vi "START_SESSION_DECODE.vi"(6 "MIMIC HOST COMMAND":T2(ring)=enum."Start Session", 8 "Input String Data Array":string[](array[string])=["1"], 9 "HWHSflag":bool, 10 "wait (ms)":u32=500, 11 "VISA resource name":refnum<visa-resource-name>="COM6") -> (0 "error out":errorcluster={"status"=FALSE, "code"=1073676294, "source"="VISA Read in MIMIC RecvCommand.vi->MIMIC Commands Rev 2.vi"}, 1 "Receive_buffer":u8[](array[numeric]) format="%x", 2 "Receive_Unpacked_Data":T1)   [LabVIEW 2014]
panel:
  out "local":i32
  out "GUID":string
  out "Array":u8[](array[numeric]) format="%x"
  out "TimeToDecode":u16
  out "VISA resource name OUT":refnum<visa-resource-name>="COM6"
  out "hex integer string":string[](array[string])=["4", "D0", "0", "0", "FF", "2C"]
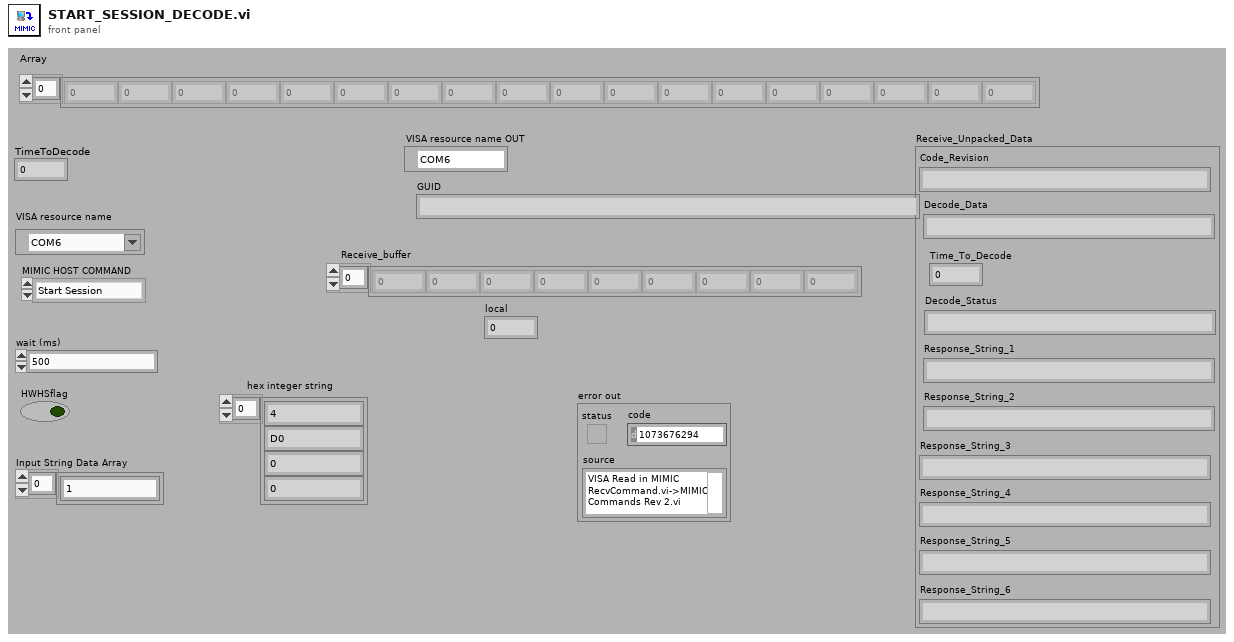
[diagram p1: front panel]
types:
  T1 = cluster{"Code_Revision":string, "Decode_Data":string, "Decode_Status":string, "Response_String_1":string, "Response_String_2":string, "Response_String_3":string, "Response_String_4":string, "Response_String_5":string, "Response_String_6":string, "Time_To_Decode":u16}
  T2 = enum16{"Enter FAT", "Beeper Control", "LED Off", "LED On", "Image Mode", "Start Session", "Stop Session", "Change Buadrate", "Auto Exposure", "Set Manual Exposure", "Read BT Address", "Store BT Address", "Pairing Command", "Query Paired Address", "Pairing Status", "Un-Pairing", "Set Illumination", "Trigger", "Set Defaults", "Imager Time To Decode Test", "Battery Off", "Battery Charge Control", "Read Battery Voltage", "Read Battery Temperature", "Software Version", "StoreFeatureSet", "ReadFeatureSet", "Store Model Number", "Read Model Number", "Store Manufacturing Date", "Read Manufacturing Date", "Store Service Date", "Read Service Date", "Store Serial Number", "Read Serial Number", "Exit FAT", "Read GUID", "Cable Auto ID", "Store RSM 627", "Read RSM 627", "Hall Effect switch", "Store GUID ", "ParamSend", "General", "General-Response", "RSM Init", "RSM EnterFAT", "RSM - SE4500 - Peek PRISM Register GENERIC command", "RSM - SE4500 - Poke PRISM Register GENERIC command", "RSM - SE4500 - GENERIC command", "RSM - SE4500 - GetPDM Calibration", "RSM - SE4500 - SetPDM Calibration", "Get Object Sensor Value", "Store Object Sensor Calibration Value", "Read Object Sensor Calibration Value", "RSM - SE4500 - GetPDM-Z Calibration", "RSM - SE4500 - SetPDM-Z Calibration"}
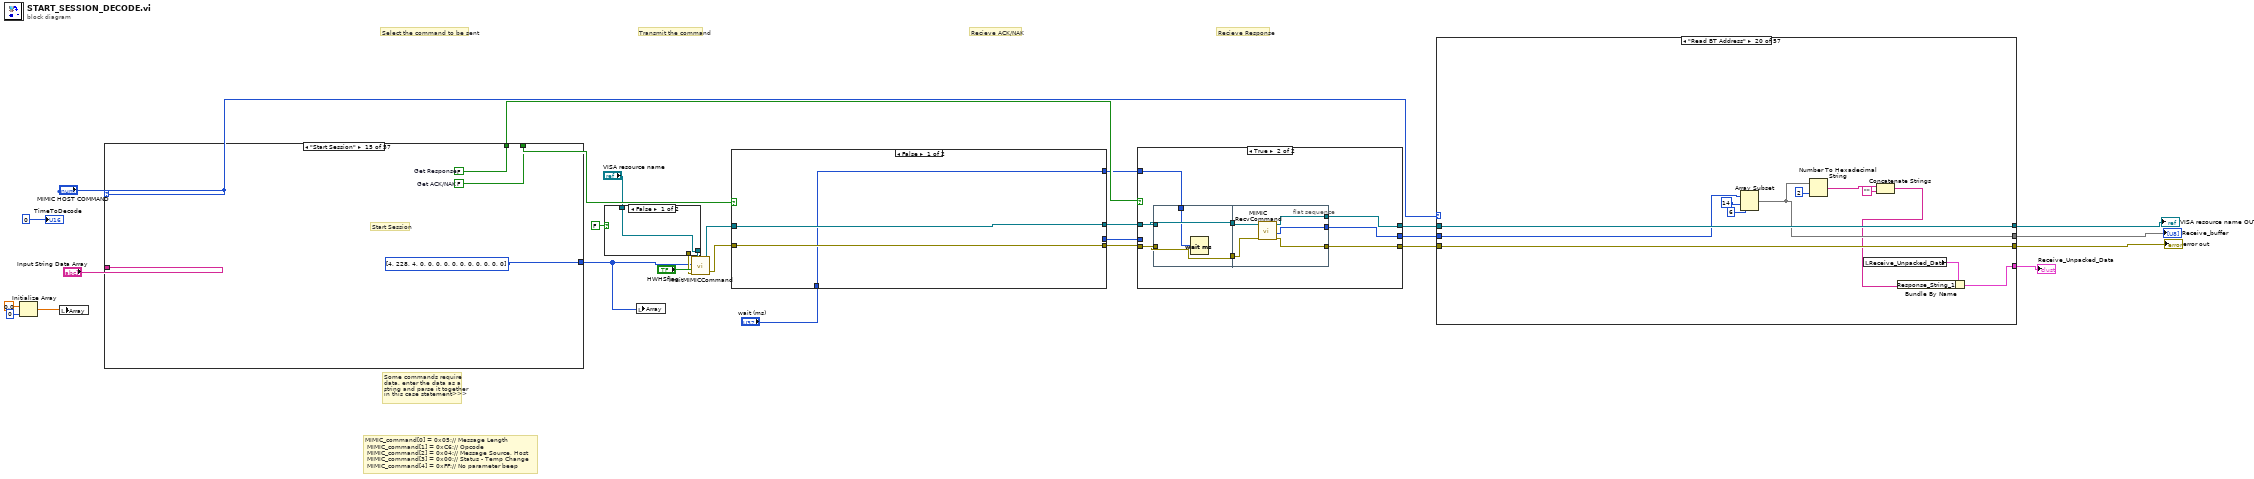
[diagram p0: block diagram]
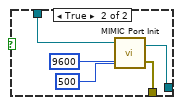
[diagram p2: hidden frame]
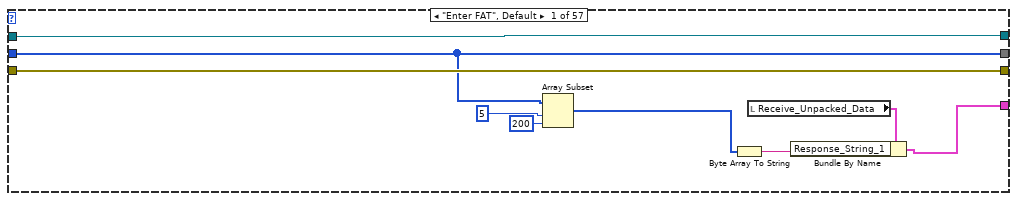
[diagram p3: hidden frame]
diagram:
  # "MIMIC_command[0] = 0x05;// Message Length \n\tMIMIC_command[1] = 0xC6;// Opcode  \n\tMIMIC_command[2] = 0x04;// Message Source, Host \n\tMIMIC_command[3] = 0x00;// Status - Temp Change            \n\tMIMIC_command[4] = 0xFF;// No parameter beep"
  # "Transmit the command"
  # "Recieve Response"
  # "Recieve ACK/NAK"
  # "Select the command to be sent"
  # "Some commands require\ndata, enter the data as a\nstring and parse it together\nin this case statement>>>"
  n1 = Initialize Array(0.0 ("element"), 0 ("dimension size")) -> (w5:dbl[])
  n2 = local write "Array"(w5) -> ()
  n3 = case shown="\"Start Session\"" "MIMIC HOST COMMAND" {
    tunnel: "Input String Data Array" -> [w37 w39 w62 _ _ _ _ _ w86 w113 w139 w179 w219 w256 _ _ _ w274 w290 w300 w313 w331 w347 _ _ _ _ _ w371 _ _ _ w391 _ _ _ _ w416 _ w428 _ w438 _ _ _ w464 _ w476 _ _ _ _ _ _ _ _ _]
    tunnel: [w31 w45 w66 u8[] [5, 161, 4, 128, 16, 0, 0, 0, 0, 0, 0, 0, 0, 0] u8[] [14, 128, 4, 0, 0, 10, 112, 0, 1, 20, 112, 12, 0, 132] u8[] [14, 128, 4, 0, 0, 10, 112, 0, 1, 20, 112, 31, 0, 113] u8[] [12, 128, 4, 0, 0, 6, 32, 0, 0, 240, 0, 0, 0, 0] u8[] [13, 128, 4, 0, 0, 9, 112, 0, 1, 2, 120, 1, 135, 0] w85 w119 w140 w176 w217 w257 u8[] [4, 228, 4, 0, 0, 0, 0, 0, 0, 0, 0, 0, 0, 0] u8[] [4, 228, 4, 0, 0, 0, 0, 0, 0, 0, 0, 0, 0, 0] u8[] [7, 215, 4, 0, 4, 11, 0, 255, 15, 0, 0, 0, 0, 0] w275 w284 w298 w317 w334 w346 u8[] [16, 161, 4, 128, 16, 0, 0, 0, 0, 0, 0, 0, 0, 0] u8[] [5, 161, 4, 128, 16, 0, 0, 0, 0, 0, 0, 0, 0, 0] u8[] [4, 200, 4, 128, 0, 0, 0, 0, 0, 0, 0, 0, 0, 0] u8[] [5, 161, 4, 128, 25, 0, 0, 0, 0, 0, 0, 0, 0, 0] u8[] [7, 161, 4, 128, 66, 2, 29, 0, 0, 0, 0, 0, 0, 0] w370 u8[] [6, 161, 4, 128, 45, 2, 0, 0, 0, 0, 0, 0, 0, 0] u8[] [7, 161, 4, 128, 48, 19, 136, 0, 0, 0, 0, 0, 0, 0] u8[] [5, 161, 4, 128, 60, 0, 0, 0, 0, 0, 0, 0, 0, 0] w390 u8[] [7, 161, 4, 128, 66, 117, 48, 0, 0, 0, 0, 0, 0, 0] u8[] [7, 161, 4, 128, 66, 117, 49, 0, 0, 0, 0, 0, 0, 0] u8[] [7, 161, 4, 128, 66, 78, 41, 0, 0, 0, 0, 0, 0, 0] u8[] [6, 161, 4, 128, 96, 8] w409 u8[] [7, 161, 4, 128, 66, 3, 36] w430 u8[] [7, 161, 4, 128, 66, 2, 194, 0, 0, 0, 0, 0, 0, 0] w443 u8[] [7, 161, 4, 128, 66, 2, 21, 0, 0, 0, 0, 0, 0, 0] w457 u8[] [7, 161, 4, 128, 66, 2, 23, 0, 0, 0, 0, 0, 0, 0] w469 u8[] [7, 161, 4, 128, 66, 2, 24, 0, 0, 0, 0, 0, 0, 0] w481 u8[] [7, 161, 4, 128, 66, 2, 22, 0, 0, 0, 0, 0, 0, 0] u8[] [5, 161, 4, 128, 54, 254, 160, 0, 0, 0, 0, 0, 0, 0] u8[] [5, 161, 4, 128, 84, 0, 0, 0, 0, 0, 0, 0, 0, 0] u8[] [5, 161, 4, 128, 47] w496 u8[] [5, 161, 4, 128, 110] u8[] [10, 161, 4, 128, 69, 2, 115, 66, 7, 2] u8[] [6, 161, 4, 128, 45, 1, 0, 0, 0, 0, 0, 0, 0, 0] u8[] [7, 161, 4, 128, 66, 2, 115]] -> w6
    tunnel: [w30 w57 w64 w71 w75 w78 w81 w84 w108 w135 w172 w192 w232 w258 w266 w269 w271 w276 w291 w301 w318 w335 w353 w356 w358 w361 w365 w369 w373 w380 w384 w387 w388 w399 w402 w404 w407 w422 w425 w433 w436 w442 w447 w456 w461 w468 w472 w479 w484 w488 w492 w493 w501 w503 w506 w509 w513] -> w25
    tunnel: [w29 w56 w65 w70 w74 w77 w80 w83 w107 w134 w171 w191 w231 w259 w267 w270 w272 w277 w292 w302 w319 w336 w354 w357 w359 w362 w364 w368 w372 w381 w383 w386 w389 w398 w401 w403 w406 w421 w424 w432 w435 w441 w448 w455 w460 w467 w473 w480 w485 w487 w491 w494 w502 w504 w507 w510 w512] -> w27
    frame "LED On" {
      w30 = FALSE  # Get Response
      w29 = TRUE  # Get ACK/NAK
      # "LED data Byte"
      n4 = Index Array(array=w37, index=0) -> (element=w36:string)
      n5 = Decimal String To Number(string=w36) -> (number=w35:i32)  [unwired: 2 in, 1 out]
      n6 = Replace Array Subset(array=u8[] [5, 231, 4, 128, 1, 0, 0, 0, 0, 0, 0, 0, 0, 0], new element=w35, index=4) -> (w31:u8[])
    }
    frame "ParamSend" {
      w57 = FALSE  # Get Response
      w56 = TRUE  # Get ACK/NAK
      n7 = Array Size(array=w39) -> (size(s)=w38:i32)
      n8 = Index Array(array=w39, index=0) -> (element=w61:string)
      n9 = Add(x=w38, y=5) -> (x+y=w43:i32)
      n10 = Hexadecimal String To Number(string=w61) -> (number=w42:u32)  [unwired: 2 in, 1 out]
      n11 = Replace Array Subset(array=u8[] [5, 198, 4, 128, 255, 0, 0, 0, 0, 0, 0, 0, 0, 0], new element=w43, index=0) -> (w54:u8[])
      n12 = Replace Array Subset(array=w54, new element=w42, index=5) -> (w50:u8[])
      n13 = Index Array(array=w39, index=2) -> (element=w49:string)
      n14 = Index Array(array=w39, index=1) -> (element=w53:string)
      n15 = Hexadecimal String To Number(string=w49) -> (number=w40:u32)  [unwired: 2 in, 1 out]
      n16 = Hexadecimal String To Number(string=w53) -> (number=w41:u32)  [unwired: 2 in, 1 out]
      n17 = Replace Array Subset(array=w50, new element=w41, index=6) -> (w46:u8[])
      n18 = Replace Array Subset(array=w46, new element=w40, index=7) -> (w45:u8[])
    }
    frame "Beeper Control" {
      w64 = FALSE  # Get Response
      w65 = TRUE  # Get ACK/NAK
      # "Beeper data Byte"
      n19 = Decimal String To Number(string=w62, offset=0) -> (number=w69:i32[])  [unwired: 1 in, 1 out]
      n20 = Replace Array Subset(array=u8[] [5, 230, 4, 128, 0, 0, 0, 0, 0, 0, 0, 0, 0, 0], new element=w69, index=4) -> (w66:u8[])
    }
    frame "Enter FAT" {
      w71 = TRUE  # Get Response
      w70 = TRUE  # Get ACK/NAK
      # "Enter FAT command:\n0x05:0xA1:0x40:0x80:0x10"
    }
    frame "RSM - SE4500 - GetPDM Calibration" {
      w75 = TRUE  # Get Response
      w74 = FALSE  # Get ACK/NAK
      # "RSM GetDPMCalibration Command"
    }
    frame "RSM - SE4500 - GetPDM-Z Calibration" {
      w78 = TRUE  # Get Response
      w77 = FALSE  # Get ACK/NAK
      # "RSM GetDPMCalibration Command"
    }
    frame "RSM Init" {
      w81 = TRUE  # Get Response
      w80 = FALSE  # Get ACK/NAK
      # "Init RSM command:\n0x0C:0x80:0x04:0x00:0x00:0x06:0x20:0x00:0x00:0xF0"
    }
    frame "RSM EnterFAT" {
      w84 = TRUE  # Get Response
      w83 = FALSE  # Get ACK/NAK
      # "RSM / SE4500 - Enter FAT command:\n0x0D:0x80:0x04:0x00:0x00:0x09:0x70:0x00:0x01:0x02:0x78:0x01:0x87:"
    }
    frame "RSM - SE4500 - Peek PRISM Register GENERIC command" {
      w108 = TRUE  # Get Response
      w107 = FALSE  # Get ACK/NAK
      # "Register Word - HEX String"
      # "RSM / SE4500 - Peek PRISM Register GENERIC command:\n0x0E:0x80:0x04:0x00:0x00:0x0B:0x70:0x00:0x01:0x02:0xC3:0xXX:0xXX:0xXX:0xCS"
      n21 = Index Array(array=w86, index=0) -> (element=w90:string)
      n22 = Hexadecimal String To Number(string=w90, default (0uL)=i16 0 ("default (0 I32)")) -> (number=w88:i16)  [unwired: 1 in, 1 out]
      n23 = Split Number(x=w88) -> (hi(x)=w94:u8, lo(x)=w92:u8)
      n24 = Replace Array Subset(array=u8[] [15, 128, 4, 0, 0, 11, 112, 0, 1, 3, 195, 0, 0, 0, 0], new element=w94, index=11) -> (w91:u8[])
      n25 = Replace Array Subset(array=w91, new element=w92, index=12) -> (w87:u8[])
      n26 = Array Subset(array=w87, index=10, length=3) -> (w97:u8[])
      n27 = for {
        N: 3 -> [_]
        tunnel: w97 -> [w111] mode=indexing
        shift-right: [w109] -> w103
        shift-left: u16 0 -> [w110]
        n28 = Add(x=w110, y=w111) -> (x+y=w109:u16)
      }
      n29 = Not(x=w103) -> (.not. x?=w102:u16)
      n30 = Increment(x=w102) -> (x+1=w101:u16)
      n31 = Replace Array Subset(array=w87, new element=w101, index=13) -> (w85:u8[])
    }
    frame "RSM - SE4500 - GENERIC command" {
      w114 = 1 ("index")
      w118 = 0 ("index")
      w135 = TRUE  # Get Response
      w134 = FALSE  # Get ACK/NAK
      # "Register Word - HEX String"
      # "RSM / SE4500 - Peek PRISM Register GENERIC command:\n0x0E:0x80:0x04:0x00:0x00:0x0B:0x70:0x00:0x01:0x02:0xXX:0xXX:0xXX:0xCS"
      n32 = Index Array(array=w113, index=w118) -> (element=w121:string)
      n33 = Index Array(array=w113, index=w114) -> (element=w115:string)
      n34 = Hexadecimal String To Number(string=w121, default (0uL)=w118) -> (number=w116:i32)  [unwired: 1 in, 1 out]
      n35 = Hexadecimal String To Number(string=w115, default (0uL)=w114) -> (number=w112:i32)  [unwired: 1 in, 1 out]
      n36 = Replace Array Subset(array=u8[] [13, 128, 4, 0, 0, 9, 112, 0, 1, 2, 255, 0, 0], new element=w116, index=10) -> (w122:u8[])
      n37 = Replace Array Subset(array=w122, new element=w112, index=11) -> (w120:u8[])
      n38 = Array Subset(array=w120, index=10, length=2) -> (w125:u8[])
      n39 = for {
        N: 2 -> [_]
        tunnel: w125 -> [w138] mode=indexing
        shift-right: [w136] -> w131
        shift-left: u16 0 -> [w137]
        n40 = Add(x=w137, y=w138) -> (x+y=w136:u16)
      }
      n41 = Not(x=w131) -> (.not. x?=w130:u16)
      n42 = Increment(x=w130) -> (x+1=w129:u16)
      n43 = Replace Array Subset(array=w120, new element=w129, index=12) -> (w119:u8[])
    }
    frame "RSM - SE4500 - Poke PRISM Register GENERIC command" {
      w172 = TRUE  # Get Response
      w171 = FALSE  # Get ACK/NAK
      # "Register Word - HEX String"
      # "Register Word - HEX String"
      # "Value Byte - Decimal String"
      # "RSM / SE4500 - Poke PRISM Register GENERIC command:\n0x0E:0x80:0x04:0x00:0x00:0x0B:0x70:0x00:0x01:0x02:0xC0:0xXX:0xXX:0xXX:0xCS"
      n44 = Index Array(array=w139, index=0) -> (element=w154:string)
      n45 = Index Array(array=w139, index=1) -> (element=w145:string)
      n46 = Hexadecimal String To Number(string=w154, default (0uL)=i16 0 ("default (0 I32)")) -> (number=w152:i16)  [unwired: 1 in, 1 out]
      n47 = Split Number(x=w152) -> (hi(x)=w158:u8, lo(x)=w156:u8)
      n48 = Hexadecimal String To Number(string=w145, default (0uL)=i16 0 ("default (0 I32)")) -> (number=w151:i16)  [unwired: 1 in, 1 out]
      n49 = Replace Array Subset(array=u8[] [16, 128, 4, 0, 0, 12, 112, 0, 1, 2, 151, 0, 0, 0, 0, 0], new element=w158, index=12) -> (w155:u8[])
      n50 = Split Number(x=w151) -> (hi(x)=w148:u8, lo(x)=w150:u8)
      n51 = Replace Array Subset(array=w155, new element=w156, index=11) -> (w143:u8[])
      n52 = Replace Array Subset(array=w143, new element=w148, index=14) -> (w142:u8[])
      n53 = Replace Array Subset(array=w142, new element=w150, index=13) -> (w141:u8[])
      n54 = Array Subset(array=w141, index=10, length=5) -> (w161:u8[])
      n55 = for {
        N: 5 -> [_]
        tunnel: w161 -> [w175] mode=indexing
        shift-right: [w173] -> w167
        shift-left: u16 0 -> [w174]
        n56 = Add(x=w174, y=w175) -> (x+y=w173:u16)
      }
      n57 = Not(x=w167) -> (.not. x?=w166:u16)
      n58 = Increment(x=w166) -> (x+1=w165:u16)
      n59 = Replace Array Subset(array=w141, new element=w165, index=15) -> (w140:u8[])
    }
    frame "RSM - SE4500 - SetPDM Calibration" {
      w192 = TRUE  # Get Response
      w191 = FALSE  # Get ACK/NAK
      # "RSM / SE4500 - SetDPMCalibration command:"
      n60 = for {
        N: 8 -> [_]
        shift-right: [w202] -> w178
        shift-left: u8[] [30, 128, 4, 0, 0, 26, 112, 0, 1, 2, 148, 12, 0, 0, 0, 0, 0, 0, 0, 0, 0, 0, 0, 0, 0, 0, 0, 0, 0, 0, 0] -> [w209]
        tunnel: w179 -> [w208]
        i -> [w204]
        # "high byte"
        # "low byte"
        n61 = Index Array(array=w208, index=w204) -> (element=w197:string)
        n62 = Decimal String To Number(string=w197, default (0L)=0 ("default (0 I32)")) -> (number=w194:i32)  [unwired: 1 in, 1 out]
        n63 = Number To Hexadecimal String(1:i16 4 ("width (-)"), 2:w194) -> (0:w195:string)
        n64 = local read "local"() -> (w200:i32)
        n65 = Hexadecimal String To Number(string=w195, default (0uL)=i16 0 ("default (0 I32)")) -> (number=w210:i16)  [unwired: 1 in, 1 out]
        n66 = Add(x=1 ("y"), y=w200) -> (x+y=w198:i32)
        n67 = Add(x=w204, y=w198) -> (x+y=w201:i32)
        n68 = Add(x=1 ("index"), y=w201) -> (x+y=w206:i32)
        n69 = Split Number(x=w210) -> (hi(x)=w212:u8, lo(x)=w211:u8)
        n70 = Replace Array Subset(array=w209, new element=w212, index=w206) -> (w203:u8[])
        n71 = local write "local"(w198) -> ()
        n72 = Replace Array Subset(array=w203, new element=w211, index=w201) -> (w202:u8[])
      }
      n73 = Array Subset(array=w178, index=10, length=19) -> (w182:u8[])
      n74 = for {
        N: 19 -> [_]
        tunnel: w182 -> [w215] mode=indexing
        shift-right: [w213] -> w188
        shift-left: u16 0 -> [w214]
        n75 = Add(x=w214, y=w215) -> (x+y=w213:u16)
      }
      n76 = Not(x=w188) -> (.not. x?=w187:u16)
      n77 = Increment(x=w187) -> (x+1=w186:u16)
      n78 = Replace Array Subset(array=w178, new element=w186, index=29) -> (w176:u8[])
      "local" <- 12 ("x+y")
    }
    frame "RSM - SE4500 - SetPDM-Z Calibration" {
      w232 = TRUE  # Get Response
      w231 = FALSE  # Get ACK/NAK
      # "RSM / SE4500 - SetDPMCalibration command:"
      n79 = local write "local"(12 ("x+y")) -> ()
      n80 = for {
        N: 8 -> [_]
        shift-right: [w242] -> w218
        shift-left: u8[] [30, 128, 4, 0, 0, 26, 112, 0, 1, 2, 148, 31, 0, 0, 0, 0, 0, 0, 0, 0, 0, 0, 0, 0, 0, 0, 0, 0, 0, 0, 0] -> [w249]
        tunnel: w219 -> [w248]
        i -> [w244]
        # "high byte"
        # "low byte"
        n81 = Index Array(array=w248, index=w244) -> (element=w237:string)
        n82 = Decimal String To Number(string=w237, default (0L)=0 ("default (0 I32)")) -> (number=w234:i32)  [unwired: 1 in, 1 out]
        n83 = Number To Hexadecimal String(1:i16 4 ("width (-)"), 2:w234) -> (0:w235:string)
        n84 = local read "local"() -> (w240:i32)
        n85 = Hexadecimal String To Number(string=w235, default (0uL)=i16 0 ("default (0 I32)")) -> (number=w250:i16)  [unwired: 1 in, 1 out]
        n86 = Add(x=1 ("y"), y=w240) -> (x+y=w238:i32)
        n87 = Add(x=w244, y=w238) -> (x+y=w241:i32)
        n88 = Add(x=1 ("index"), y=w241) -> (x+y=w246:i32)
        n89 = Split Number(x=w250) -> (hi(x)=w252:u8, lo(x)=w251:u8)
        n90 = Replace Array Subset(array=w249, new element=w252, index=w246) -> (w243:u8[])
        n91 = local write "local"(w238) -> ()
        n92 = Replace Array Subset(array=w243, new element=w251, index=w241) -> (w242:u8[])
      }
      n93 = Array Subset(array=w218, index=10, length=19) -> (w222:u8[])
      n94 = for {
        N: 19 -> [_]
        tunnel: w222 -> [w255] mode=indexing
        shift-right: [w253] -> w228
        shift-left: u16 0 -> [w254]
        n95 = Add(x=w254, y=w255) -> (x+y=w253:u16)
      }
      n96 = Not(x=w228) -> (.not. x?=w227:u16)
      n97 = Increment(x=w227) -> (x+1=w226:u16)
      n98 = Replace Array Subset(array=w218, new element=w226, index=29) -> (w217:u8[])
    }
    frame "Image Mode" {
      w258 = FALSE  # Get Response
      w259 = TRUE  # Get ACK/NAK
      # "Image Mode Byte:\n00: Decode\n01: SnapShot\n02: Video\n03: Last Decode\n04: las No Decode"
      n99 = Index Array(array=w256, index=0) -> (element=w264:string)
      n100 = Decimal String To Number(string=w264) -> (number=w263:i32)  [unwired: 2 in, 1 out]
      n101 = Replace Array Subset(array=u8[] [5, 247, 4, 128, 0, 0, 0, 0, 0, 0, 0, 0, 0, 0], new element=w263, index=4) -> (w257:u8[])
    }
    frame "Start Session" {
      w266 = FALSE  # Get Response
      w267 = FALSE  # Get ACK/NAK
      # "Start Session"
    }
    frame "Stop Session" {
      w269 = FALSE  # Get Response
      w270 = TRUE  # Get ACK/NAK
      # "Start Session"
    }
    frame "Change Buadrate" {
      w271 = FALSE  # Get Response
      w272 = FALSE  # Get ACK/NAK
      # "Enter FAT command:\n06: 9600\n08: 38400\n0A: 57600\n0B:115200\n0C:230400"
    }
    frame "Auto Exposure" {
      w276 = FALSE  # Get Response
      w277 = TRUE  # Get ACK/NAK
      # "Auto Exposure:\n00:Disabled\n01: Enabled"
      n102 = Index Array(array=w274, index=0) -> (element=w282:string)
      n103 = Decimal String To Number(string=w282) -> (number=w281:i32)  [unwired: 2 in, 1 out]
      n104 = Replace Array Subset(array=u8[] [8, 198, 4, 0, 255, 240, 41, 0, 0, 0, 0, 0, 0, 0], new element=w281, index=7) -> (w275:u8[])
    }
    frame "Set Manual Exposure" {
      w291 = FALSE  # Get Response
      w292 = TRUE  # Get ACK/NAK
      # "Image Mode Byte:\n00: Decode\n01: SnapShot\n02: Video\n03: Last Decode\n04: las No Decode"
      n105 = Index Array(array=w290, index=0) -> (element=w296:string)
      n106 = Decimal String To Number(string=w296, default (0L)=u16 0 ("default (0 I32)")) -> (number=w289:u16)  [unwired: 1 in, 1 out]
      n107 = Split Number(x=w289) -> (hi(x)=w287:u8, lo(x)=w286:u8)
      n108 = Replace Array Subset(array=u8[] [10, 198, 4, 0, 255, 244, 241, 55, 0, 0, 0, 0, 0, 0], new element=w287, index=8) -> (w283:u8[])
      n109 = Replace Array Subset(array=w283, new element=w286, index=9) -> (w284:u8[])
    }
    frame "Store BT Address" {
      w301 = FALSE  # Get Response
      w302 = TRUE  # Get ACK/NAK
      # "Store BT command:\n0x16, 0xA1, 0x04, 0x80, 0x45, 0x02, 0x1D, 0x41, 0x07, 0x42, 0x00, 0x06, 0x00, 0x00, \n\t\t\t\t\t\t\t\t\t\t0x00, 0x00, 0x00, 0x00, 0x00, 0x00,0x00, 0x00, 0xFF, 0xFF};"
      n110 = for {
        N: 6 -> [_]
        tunnel: w300 -> [w311]
        tunnel: [w306] -> w298
        i -> [w308]
        n111 = Index Array(array=w311, index=w308) -> (element=w305:string)
        n112 = Add(x=14 ("index"), y=w308) -> (x+y=w309:i32)
        n113 = Hexadecimal String To Number(string=w305, offset=0) -> (number=w303:u32)  [unwired: 1 in, 1 out]
        n114 = local read "Array"() -> (w307:u8[])
        n115 = Replace Array Subset(array=w307, new element=w303, index=w309) -> (w306:u8[])
        n116 = local write "Array"(w306) -> ()
      }
      "Array" <- u8[] [22, 161, 4, 128, 69, 2, 29, 65, 7, 66, 0, 6, 0, 0, 0, 0, 0, 0, 0, 0, 255, 255, 255, 0, 0, 0]
    }
    frame "General" {
      w315 = 0 ("offset")
      w318 = FALSE  # Get Response
      w319 = TRUE  # Get ACK/NAK
      # "Gneral FAT command:\n0x16, 0xA1, 0x04, 0x80, 0x45, 0x02, 0x1D, 0x41, 0x07, 0x42, 0x00, 0x06, 0x00, 0x00, \n\t\t\t\t\t\t\t\t\t\t0x00, 0x00, 0x00, 0x00, 0x00, 0x00,0x00, 0x00, 0xFF, 0xFF};"
      n117 = Index Array(array=w313, index=w315) -> (element=w314:string)
      n118 = Hexadecimal String To Number(string=w314, offset=w315) -> (number=w312:u32)  [unwired: 1 in, 1 out]
      n119 = for {
        N: w312 -> [_]
        tunnel: w313 -> [w328]
        tunnel: [w323] -> w317
        i -> [w325]
        n120 = Index Array(array=w328, index=w325) -> (element=w322:string)
        n121 = Add(x=0 ("index"), y=w325) -> (x+y=w326:i32)
        n122 = Hexadecimal String To Number(string=w322, offset=0) -> (number=w320:u32)  [unwired: 1 in, 1 out]
        n123 = local read "Array"() -> (w324:u8[])
        n124 = Replace Array Subset(array=w324, new element=w320, index=w326) -> (w323:u8[])
        n125 = local write "Array"(w323) -> ()
      }
      n126 = local write "Array"(u8[] [22, 0, 0, 0, 0, 0, 0, 0, 0, 0, 0, 0, 0, 0, 0, 0, 0, 0, 0, 0, 0, 0, 0, 0, 0, 0]) -> ()
    }
    frame "General-Response" {
      w330 = 0 ("offset")
      w335 = TRUE  # Get Response
      w336 = TRUE  # Get ACK/NAK
      # "Gneral FAT command:\n0x16, 0xA1, 0x04, 0x80, 0x45, 0x02, 0x1D, 0x41, 0x07, 0x42, 0x00, 0x06, 0x00, 0x00, \n\t\t\t\t\t\t\t\t\t\t0x00, 0x00, 0x00, 0x00, 0x00, 0x00,0x00, 0x00, 0xFF, 0xFF};"
      n127 = Index Array(array=w331, index=w330) -> (element=w329:string)
      n128 = Hexadecimal String To Number(string=w329, offset=w330) -> (number=w332:u32)  [unwired: 1 in, 1 out]
      n129 = for {
        N: w332 -> [_]
        tunnel: w331 -> [w345]
        tunnel: [w340] -> w334
        i -> [w342]
        n130 = Index Array(array=w345, index=w342) -> (element=w339:string)
        n131 = Add(x=0 ("index"), y=w342) -> (x+y=w343:i32)
        n132 = Hexadecimal String To Number(string=w339, offset=0) -> (number=w337:u32)  [unwired: 1 in, 1 out]
        n133 = local read "Array"() -> (w341:u8[])
        n134 = Replace Array Subset(array=w341, new element=w337, index=w343) -> (w340:u8[])
        n135 = local write "Array"(w340) -> ()
      }
      n136 = local write "Array"(u8[] [22, 0, 0, 0, 0, 0, 0, 0, 0, 0, 0, 0, 0, 0, 0, 0, 0, 0, 0, 0, 0, 0, 0, 0, 0, 0]) -> ()
    }
    frame "Pairing Command" {
      w353 = TRUE  # Get Response
      w354 = FALSE  # Get ACK/NAK
      # "Pairing  command:\n10 9E 04 80 00 00 02 03 06 08  01 0B 03 00 0F 0F FE 8E"
      n137 = Index Array(array=w347, index=0) -> (element=w351:string)
      n138 = String To Byte Array(string=w351) -> (unsigned byte array=w349:u8[])
      n139 = Replace Array Subset(array=u8[] [16, 158, 4, 128, 0, 0, 0, 0, 0, 8, 1, 11, 3, 0, 15, 15], new element=w349, index=4) -> (w346:u8[])
    }
    frame "Un-Pairing" {
      w356 = TRUE  # Get Response
      w357 = FALSE  # Get ACK/NAK
      # "Enter FAT command:\n0x05:0xA1:0x40:0x80:0x10"
    }
    frame "Set Illumination" {
      w358 = TRUE  # Get Response
      w359 = FALSE  # Get ACK/NAK
      # "Enter FAT command:\n0x05:0xA1:0x40:0x80:0x10"
    }
    frame "Set Defaults" {
      w361 = FALSE  # Get Response
      w362 = TRUE  # Get ACK/NAK
    }
    frame "Exit FAT" {
      w365 = TRUE  # Get Response
      w364 = TRUE  # Get ACK/NAK
    }
    frame "Read BT Address" {
      w369 = TRUE  # Get Response
      w368 = TRUE  # Get ACK/NAK
    }
    frame "LED Off" {
      w373 = FALSE  # Get Response
      w372 = TRUE  # Get ACK/NAK
      # "LED data Byte"
      n140 = Index Array(array=w371, index=0) -> (element=w378:string)
      n141 = Decimal String To Number(string=w378) -> (number=w377:i32)  [unwired: 2 in, 1 out]
      n142 = Replace Array Subset(array=u8[] [5, 232, 4, 128, 1, 0, 0, 0, 0, 0, 0, 0, 0, 0], new element=w377, index=4) -> (w370:u8[])
    }
    frame "Trigger" {
      w380 = TRUE  # Get Response
      w381 = TRUE  # Get ACK/NAK
    }
    frame "Imager Time To Decode Test" {
      w384 = TRUE  # Get Response
      w383 = TRUE  # Get ACK/NAK
      # "Start Session"
    }
    frame "Battery Off" {
      w387 = FALSE  # Get Response
      w386 = TRUE  # Get ACK/NAK
      # "Enter FAT command:\n0x05:0xA1:0x40:0x80:0x10"
    }
    frame "Battery Charge Control" {
      w388 = FALSE  # Get Response
      w389 = TRUE  # Get ACK/NAK
      # "Battery Charge\n0x06, 0xA1, 0x04, 0x80, 0x3D\n0x00: Disable charging of battery\n0x01: Enable charging of battery\n0x02: Enable Slow charge (Hammer)"
      n143 = Index Array(array=w391, index=0) -> (element=w396:string)
      n144 = Decimal String To Number(string=w396) -> (number=w395:i32)  [unwired: 2 in, 1 out]
      n145 = Replace Array Subset(array=u8[] [6, 161, 4, 128, 61, 0, 0, 0, 0, 0, 0, 0, 0, 0], new element=w395, index=5) -> (w390:u8[])
    }
    frame "Read Battery Voltage" {
      w399 = TRUE  # Get Response
      w398 = FALSE  # Get ACK/NAK
      # "Read Battery Voltage command:\n0x07:0xA1:0x04:0x80:0x42:0x75:0x30"
    }
    frame "Read Battery Temperature" {
      w402 = TRUE  # Get Response
      w401 = FALSE  # Get ACK/NAK
      # "Read Battery Temperature command:\n0x07:0xA1:0x04:0x80:0x42:0x75:0x31"
    }
    frame "Software Version" {
      w404 = TRUE  # Get Response
      w403 = TRUE  # Get ACK/NAK
      # "Software Version command:\n\"0x07, 0xA1, 0x04, 0x80, 0x42, 0x4E, 0x29,\""
    }
    frame "Get Object Sensor Value" {
      w407 = TRUE  # Get Response
      w406 = TRUE  # Get ACK/NAK
      # "Get Object Sensor command:\n\"0x06,0xA1,0x04,0x80,0x60,0x08,\""
    }
    frame "Store Object Sensor Calibration Value" {
      w422 = FALSE  # Get Response
      w421 = TRUE  # Get ACK/NAK
      # "Store Object Sensor Calibration command:\n\"0x0B,0xA1,0x04,0x80,0x45,0x03,0x24,0x57,0x07,CAL H,CAL L"
      n146 = Index Array(array=w416, index=1) -> (element=w411:string)
      n147 = Index Array(array=w416, index=0) -> (element=w419:string)
      n148 = Hexadecimal String To Number(string=w419) -> (number=w412:u32)  [unwired: 2 in, 1 out]
      n149 = Hexadecimal String To Number(string=w411) -> (number=w410:u32)  [unwired: 2 in, 1 out]
      n150 = Replace Array Subset(array=u8[] [11, 161, 4, 128, 69, 3, 36, 87, 7, 0, 0], new element=w412, index=9) -> (w414:u8[])
      n151 = Replace Array Subset(array=w414, new element=w410, index=10) -> (w409:u8[])
    }
    frame "Read Object Sensor Calibration Value" {
      w425 = TRUE  # Get Response
      w424 = TRUE  # Get ACK/NAK
      # "Read Object Sensor Calibration command:\n\"0x07,0xA1,0x04,0x80,0x42,0x03,0x24,\""
    }
    frame "StoreFeatureSet" {
      w433 = FALSE  # Get Response
      w432 = TRUE  # Get ACK/NAK
      # "Store Feature Set command:\n\"0x0A, 0xA1, 0x04, 0x80, 0x45, 0x02, 0xC2, 0x42, 0x07,\n0xFF,//Feature Set Value \n0x00, 0x00}; //checksum\""
      n152 = Hexadecimal String To Number(string=w428, offset=0) -> (number=w426:u32[])  [unwired: 1 in, 1 out]
      n153 = Replace Array Subset(array=u8[] [10, 161, 4, 128, 69, 2, 194, 66, 7, 0, 0, 0, 0, 0], new element=w426, index=9) -> (w430:u8[])
    }
    frame "ReadFeatureSet" {
      w436 = TRUE  # Get Response
      w435 = TRUE  # Get ACK/NAK
      # "0x07, 0xA1, 0x04, 0x80, 0x42, 0x02, 0xC2, 0x00, 0x00};"
      # "Read Feature Set command:\n0x07, 0xA1, 0x04, 0x80, 0x42, 0x02, 0xC2,"
    }
    frame "Store Model Number" {
      w442 = FALSE  # Get Response
      w441 = TRUE  # Get ACK/NAK
      # "StoreModel Number command:\n0x20, 0xA1, 0x04, 0x80, 0x45, 0x02, 0x15, 0x53, 0x07, 0x00, 0x12, 0x00, 0x00,\n\t\t\t\t\t\t\t\t\t\t0x00, 0x00, 0x00, 0x00, 0x00, 0x00, 0x00, 0x00, 0x00,\n\t\t\t\t\t\t\t\t\t\t0x00, 0x00, 0x00, 0x00, 0x00, 0x00, 0x00, 0x00, 0x00,\n\t\t\t\t\t\t\t\t\t\t0x00"
      n154 = Index Array(array=w438, index=0) -> (element=w439:string)
      n155 = String To Byte Array(string=w439) -> (unsigned byte array=w440:u8[])
      n156 = Replace Array Subset(array=u8[] [32, 161, 4, 128, 69, 2, 21, 83, 7, 0, 18, 0, 0, 0, 0, 0, 0, 0, 0, 0, 0, 0, 0, 0, 0, 0, 0, 0, 0, 0, 0, 0, 0], new element=w440, index=13) -> (w443:u8[])
    }
    frame "Read Model Number" {
      w447 = TRUE  # Get Response
      w448 = TRUE  # Get ACK/NAK
      # "ReadModel Number command:\n0x07, 0xA1, 0x04, 0x80, 0x42, 0x02, 0x15,"
    }
    frame "Store Manufacturing Date" {
      w456 = FALSE  # Get Response
      w455 = TRUE  # Get ACK/NAK
      # "Store Manufacturing Date command:\n0x15, 0xA1, 0x04, 0x80, 0x45, 0x02, 0x17, 0x53, 0x07, 0x00, 0x07, 0x00, 0x00,\n\t\t\t\t\t\t\t\t\t\t0x00, 0x00, 0x00, 0x00, 0x00, 0x00, 0x00,\n\t\t\t\t\t\t\t\t\t\t0x00"
      n157 = Get Date/Time In Seconds() -> (seconds since 1Jan1904=w454:timestamp)
      n158 = Format Date/Time String(time format string (%c)="%d%b%y", seconds (now)=w454, UTC format=FALSE) -> (date/time string=w450:string)
      n159 = To Upper Case(1:w450) -> (0:w449:string)
      n160 = String To Byte Array(string=w449) -> (unsigned byte array=w451:u8[])
      n161 = Replace Array Subset(array=u8[] [21, 161, 4, 128, 69, 2, 23, 83, 7, 0, 7, 0, 0, 0, 0, 0, 0, 0, 0, 0, 0, 0], new element=w451, index=13) -> (w457:u8[])
    }
    frame "Read Manufacturing Date" {
      w461 = TRUE  # Get Response
      w460 = TRUE  # Get ACK/NAK
      # "Read Feature Set command:\n0x07, 0xA1, 0x04, 0x80, 0x42, 0x02, 0x17,"
    }
    frame "Store Service Date" {
      w468 = FALSE  # Get Response
      w467 = TRUE  # Get ACK/NAK
      # "StoreService Date command:\n0x15, 0xA1, 0x04, 0x80, 0x45, 0x02, 0x18, 0x53, 0x07, 0x00, 0x07, 0x00, 0x00,\n\t\t\t\t\t\t\t\t\t\t0x00, 0x00, 0x00, 0x00, 0x00, 0x00, 0x00,\n\t\t\t\t\t\t\t\t\t\t0x00"
      n162 = Index Array(array=w464, index=0) -> (element=w466:string)
      n163 = String To Byte Array(string=w466) -> (unsigned byte array=w463:u8[])
      n164 = Replace Array Subset(array=u8[] [21, 161, 4, 128, 69, 2, 24, 83, 7, 0, 7, 0, 0, 0, 0, 0, 0, 0, 0, 0, 0, 0], new element=w463, index=13) -> (w469:u8[])
    }
    frame "Read Service Date" {
      w472 = TRUE  # Get Response
      w473 = TRUE  # Get ACK/NAK
      # "Read Service Date command:\n0x07, 0xA1, 0x04, 0x80, 0x42, 0x02, 0x18,"
    }
    frame "Store Serial Number" {
      w479 = FALSE  # Get Response
      w480 = TRUE  # Get ACK/NAK
      # "Store Serial Number command:\n0x1E, 0xA1, 0x04, 0x80, 0x45, 0x02, 0x16, 0x53, 0x07, 0x00, 0x10, 0x00, 0x00,\n\t\t\t\t\t\t\t\t\t\t0x00, 0x00, 0x00, 0x00, 0x00, 0x00, 0x00, 0x00,\n\t\t\t\t\t\t\t\t\t\t0x00, 0x00, 0x00, 0x00, 0x00, 0x00, 0x00, 0x00,\n\t\t\t\t\t\t\t\t\t\t0x00"
      n165 = Index Array(array=w476, index=0) -> (element=w478:string)
      n166 = String To Byte Array(string=w478) -> (unsigned byte array=w475:u8[])
      n167 = Replace Array Subset(array=u8[] [30, 161, 4, 128, 69, 2, 22, 83, 7, 0, 16, 0, 0, 0, 0, 0, 0, 0, 0, 0, 0, 0, 0, 0, 0, 0, 0, 0, 0, 0, 0, 0, 0], new element=w475, index=13) -> (w481:u8[])
    }
    frame "Read Serial Number" {
      w484 = TRUE  # Get Response
      w485 = TRUE  # Get ACK/NAK
      # "Read Serial Number command:\n0x07, 0xA1, 0x04, 0x80, 0x42, 0x02, 0x16,"
    }
    frame "Pairing Status" {
      w488 = TRUE  # Get Response
      w487 = FALSE  # Get ACK/NAK
      # "Read Serial Number command:\n0x05, 0xA1, 0x04, 0x80, 0x36, 0xFE, 0xA0,"
    }
    frame "Query Paired Address" {
      w492 = TRUE  # Get Response
      w491 = FALSE  # Get ACK/NAK
      # "Read Serial Number command:\n0x05, 0xA1, 0x04, 0x80, 0x54,"
    }
    frame "Read GUID" {
      w493 = TRUE  # Get Response
      w494 = TRUE  # Get ACK/NAK
      # "\"0x05, 0xA1, 0x04, 0x80, 0x2F,\""
    }
    frame "Store GUID " {
      w501 = TRUE  # Get Response
      w502 = FALSE  # Get ACK/NAK
      # "32 bytes 0-9, A-F (0x30 - 0x3F, 0x41 - 0x46)"
      # "Start of Date Bytes"
      # "Store GIUD command:\n0x29:0x80:0x04:0x80:0x00:0x25:0x64:0x00:0x0B:0xXX:0xXX:0xXX:0xXX:0xXX:0xXX:0xXX:0xXX:0xXX:0xXX:0xXX:0xXX:0xXX:0xXX:0xXX:0xXX:0xXX:0xXX:0xXX:0xXX:0xXX:0xXX:0xXX:0xXX:0xXX:0xXX:0xXX:0xXX:0xXX:0xXX:0xXX:0xXX:"
      n168 = call "Generate GUID.vi"() -> ("GUID"=w500:string)  [unwired: 10 in, 1 out]
      "GUID" <- w500
      n169 = String To Byte Array(string=w500) -> (unsigned byte array=w497:u8[])
      n170 = Insert Into Array(array=u8[] [41, 128, 4, 128, 0, 37, 100, 0, 11], index=9, new element=w497) -> (w496:u8[])
    }
    frame "Cable Auto ID" {
      w503 = TRUE  # Get Response
      w504 = TRUE  # Get ACK/NAK
      # "0x05, 0xA1, 0x04, 0x00, 0x6E"
    }
    frame "Store RSM 627" {
      w506 = FALSE  # Get Response
      w507 = TRUE  # Get ACK/NAK
      # "0x0A, 0xA1, 0x04, 0x80, 0x45, 0x02, 0x73, 0x42, 0x07, 0x02"
    }
    frame "Hall Effect switch" {
      w509 = TRUE  # Get Response
      w510 = TRUE  # Get ACK/NAK
    }
    frame "Read RSM 627" {
      w513 = TRUE  # Get Response
      w512 = TRUE  # Get ACK/NAK
      # "\"0x07, 0xA1, 0x04, 0x80, 0x42,0x02,0x73\""
    }
  }
  n171 = case shown="False" FALSE {
    tunnel: [w515 w519] -> w8
    tunnel: [_ w518] -> w7
    tunnel: "VISA resource name" -> [w515 w516]
    frame False {
    }
    frame True {
      n172 = call "MIMIC Port Init.vi"("MIMIC TIMEOUT"=u32 500, "MIMC BAUD"=u32 9600, "MIMIC_PORT"=w516) -> ("error out"=w518:errorcluster, "MIMIC PORT RESOURCE"=w519:refnum<visa-resource-name>)
    }
  }
  n173 = local write "Array"(w6) -> ()
  n174 = call "XmitMIMICCommand.vi"("error in (no error)"=w7, "HWHSflag"="HWHSflag", "Command array"=w6, "VISA resource name"=w8) -> ("error out"=w22:errorcluster, "VISA resource name Out"=w21:refnum<visa-resource-name>)
  n175 = case shown="False" w27 {
    tunnel: [w523 w527] -> w26
    tunnel: w22 -> [w523 w532]
    tunnel: w21 -> [w522 w530]
    tunnel: [w522 w528] -> w24
    tunnel: [_ w526] -> w16
    tunnel: [w521 w525] -> w15
    tunnel: "wait (ms)" -> [w521 w524]
    frame False {
    }
    frame True {
      # "NEED TO CHECK ACK"
      n176 = flat-sequence {
        tunnel: w532 -> [w535]
        tunnel: [w535] -> w531
        tunnel: w530 -> [w534]
        tunnel: [w534] -> w529
        tunnel: [w533] -> w525
        tunnel: w524 -> [w533]
        tunnel: w531 -> [w540]
        tunnel: w529 -> [w539]
        tunnel: [w538] -> w528
        tunnel: [w537] -> w527
        tunnel: [w536] -> w526
        frame #0 {
          n177 = Wait (ms)(milliseconds to wait=w533) -> ()  [unwired: 1 out]
        }
        frame #1 {
          n178 = call "MIMIC RecvCommand.vi"("error in"=w540, "VISA resource name"=w539) -> ("error out"=w537:errorcluster, "Receive_buffer"=w536:u8[], "VISA resource name OUT"=w538:refnum<visa-resource-name>)  [unwired: 2 in, 1 out]
          n179 = Number To Hexadecimal String(2:w536) -> (0:→"hex integer string":string[])  [unwired: 1 in]
        }
      }
    }
  }
  n180 = case shown="True" w25 {
    tunnel: [w544 w551] -> w17
    tunnel: w26 -> [w544 w546]
    tunnel: w24 -> [w543 w548]
    tunnel: [w542 w552] -> w18
    tunnel: [w543 w550] -> w19
    tunnel: w16 -> [w542 _]
    tunnel: w15 -> [_ w545]
    frame False {
    }
    frame True {
      n181 = flat-sequence {
        tunnel: [w555] -> w549
        tunnel: w548 -> [w555]
        tunnel: [w554] -> w547
        tunnel: w546 -> [w554]
        tunnel: w545 -> [w553]
        tunnel: [w560] -> w552
        tunnel: [w559] -> w551
        tunnel: [w558] -> w550
        tunnel: w549 -> [w556]
        tunnel: w547 -> [w557]
        frame #0 {
          n182 = Wait (ms)(milliseconds to wait=w553) -> ()  [unwired: 1 out]
        }
        frame #1 {
          n183 = call "MIMIC RecvCommand.vi"("error in"=w557, "VISA resource name"=w556) -> ("error out"=w559:errorcluster, "Receive_buffer"=w560:u8[], "VISA resource name OUT"=w558:refnum<visa-resource-name>)  [unwired: 2 in, 1 out]
        }
      }
    }
  }
  n184 = case shown="\"Read BT Address\"" "MIMIC HOST COMMAND" {
    tunnel: w19 -> [w568 w572 w575 w578 w581 w584 w587 w590 w593 w596 w599 w602 w605 w608 w611 w614 w617 w620 w623 w635 w638 w641 w644 w647 w650 w659 w662 w669 w688 w711 w714 w720 w756 w792 w806 w820 w823 w825 w842 w847 w850 w854 w864 w875 w883 w886 w895 w897 w908 w919 w924 w942 w945 w948 w951 w956 w969]
    tunnel: [w568 w572 w575 w578 w581 w584 w587 w590 w593 w596 w599 w602 w605 w608 w611 w614 w617 w620 w623 w635 w638 w641 w644 w647 w650 w659 w662 w669 w688 w711 w714 w720 w756 w792 w806 w820 w823 w825 w842 w847 w850 w854 w864 w875 w883 w886 w895 w897 w908 w919 w924 w942 w945 w948 w951 w956 w969] -> w13
    tunnel: w18 -> [w564 w571 w574 w577 w580 w583 w586 w589 w592 w595 w598 w601 w604 w607 w610 w613 w616 w619 w622 w633 w637 w640 w643 w646 w649 w651 w661 w664 w686 w710 w713 w716 w725 w761 w797 w811 w821 w827 w837 w846 w851 w855 w861 w874 w880 w885 w892 w898 w904 w912 w921 w937 w944 w947 w950 w953 w968]
    tunnel: [w564 w571 w574 w577 w580 w583 w586 w589 w592 w595 w598 w601 w604 w607 w610 w613 w616 w619 w622 w628 w637 w640 w643 w646 w649 w651 w661 w663 w686 w710 w713 w715 w725 w761 w797 w811 w821 w826 w840 w846 w848 w855 w859 w874 w877 w885 w890 w898 w900 w910 w923 w936 w944 w947 w950 w952 w968] -> w12
    tunnel: w17 -> [w569 w570 w573 w576 w579 w582 w585 w588 w591 w594 w597 w600 w603 w606 w609 w612 w615 w618 w621 w634 w636 w639 w642 w645 w648 w658 w660 w668 w689 w709 w712 w719 w755 w791 w805 w819 w822 w824 w841 w845 w849 w856 w865 w873 w884 w887 w896 w899 w907 w920 w925 w941 w943 w946 w949 w955 w967]
    tunnel: [w569 w570 w573 w576 w579 w582 w585 w588 w591 w594 w597 w600 w603 w606 w609 w612 w615 w618 w621 w634 w636 w639 w642 w645 w648 w658 w660 w668 w689 w709 w712 w719 w755 w791 w805 w819 w822 w824 w841 w845 w849 w856 w865 w873 w884 w887 w896 w899 w907 w920 w925 w941 w943 w946 w949 w955 w967] -> w11
    tunnel: [w566 _ _ _ _ _ _ _ _ _ _ _ _ _ _ _ _ _ _ w629 _ _ _ _ _ w655 _ _ w691 _ _ _ w726 w762 w793 w807 _ _ w838 _ _ _ w857 w867 w878 _ w888 _ w902 w911 _ w934 _ _ _ _ _] -> w9
    frame "Enter FAT", Default {
      n185 = Array Subset(array=w564, index=5, length=200) -> (w563:u8[])
      n186 = Byte Array To String(unsigned byte array=w563) -> (string=w567:string)
      n187 = local read "Receive_Unpacked_Data"() -> (w565:T1)
      n188 = Bundle By Name(cluster=w565, "Response_String_1"=w567) -> (w566:T1)
    }
    frame "Beeper Control" {
    }
    frame "ParamSend" {
    }
    frame "General" {
    }
    frame "General-Response" {
    }
    frame "RSM Init" {
    }
    frame "RSM EnterFAT" {
    }
    frame "RSM - SE4500 - Peek PRISM Register GENERIC command" {
    }
    frame "RSM - SE4500 - Poke PRISM Register GENERIC command" {
    }
    frame "RSM - SE4500 - GENERIC command" {
    }
    frame "RSM - SE4500 - SetPDM Calibration" {
    }
    frame "RSM - SE4500 - SetPDM-Z Calibration" {
    }
    frame "LED On" {
    }
    frame "Image Mode" {
    }
    frame "Start Session" {
    }
    frame "Stop Session" {
    }
    frame "Change Buadrate" {
    }
    frame "Auto Exposure" {
    }
    frame "Set Manual Exposure" {
    }
    frame "Read BT Address" {
      n189 = Array Subset(array=w633, index=14, length=6) -> (w628:u8[])
      n190 = Number To Hexadecimal String(1:i16 2 ("width (-)"), 2:w628) -> (0:w626:string[])
      n191 = local read "Receive_Unpacked_Data"() -> (w630:T1)
      n192 = Concatenate Strings(w626, "" ("string")) -> (w625:string)
      n193 = Bundle By Name(cluster=w630, "Response_String_1"=w625) -> (w629:T1)
    }
    frame "Store BT Address" {
    }
    frame "Pairing Command" {
    }
    frame "Un-Pairing" {
    }
    frame "Set Illumination" {
    }
    frame "Set Defaults" {
    }
    frame "Exit FAT" {
      n194 = Array Subset(array=w651, index=5, length=13) -> (w652:u8[])
      n195 = Byte Array To String(unsigned byte array=w652) -> (string=w657:string)
      n196 = local read "Receive_Unpacked_Data"() -> (w656:T1)
      n197 = Bundle By Name(cluster=w656, "Response_String_1"=w657) -> (w655:T1)
    }
    frame "LED Off" {
    }
    frame "Trigger" {
      n198 = Empty Array?(array=w664) -> (empty?=w665:bool)
      n199 = case shown="False" w665 {
        tunnel: w664 -> [w671 _]
        tunnel: [w670 w677] -> w663
        frame False {
          n200 = Array Subset(array=w671, index=5, length=1) -> (w670:u8[])
        }
        frame True {
          # "If empty, init array and set its values to zero."
          n201 = To Unsigned Byte Integer(number=u8 0) -> (unsigned 8bit integer=w675:u8)
          n202 = Initialize Array(w675, 1 ("dimension size")) -> (w677:u8[])
        }
      }
      n203 = Array Subset(array=w664, index=5, length=1) -> ()  [unwired: 1 out]
    }
    frame "Imager Time To Decode Test" {
      n204 = Byte Array To String(unsigned byte array=w686) -> (string=w702:string)
      n205 = Replace Substring(2:17 ("length (len. of substring)"), 3:0 ("offset (0)"), 5:w702) -> (1:w697:string)  [unwired: 1 in, 1 out]
      n206 = String Length(string=w697) -> (length=w696:i32)
      n207 = Index Array(array=w686, index=5) -> (element=w699:u8)
      n208 = Subtract(x=w696, y=2) -> (x-y=w694:i32)
      n209 = Index Array(array=w686, index=7 ("length")) -> (element=w681:u8)
      n210 = Index Array(array=w686, index=6) -> (element=w684:u8)
      n211 = case shown="1" w699 {
        frame 0, Default {
          n212 = local read "Receive_Unpacked_Data"() -> (w703:T1)
          n213 = Bundle By Name(cluster=w703, "Decode_Status"="No Decode" ("Decode_Data")) -> (w704:T1)
          n214 = local write "Receive_Unpacked_Data"(w704) -> ()
        }
        frame 1 {
          n215 = local read "Receive_Unpacked_Data"() -> (w707:T1)
          n216 = Bundle By Name(cluster=w707, "Decode_Status"="SUCCESS" ("Decode_Data")) -> (w706:T1)
          n217 = local write "Receive_Unpacked_Data"(w706) -> ()
        }
      }
      n218 = Join Numbers(hi=u8 0, lo=w684) -> ((hi.lo)=w679:u16)
      n219 = Join Numbers(hi=w681, lo=u8 0 ("hi")) -> ((hi.lo)=w680:u16)
      n220 = Add(x=w679, y=w680) -> (x+y=w678:u16)
      n221 = local write "TimeToDecode"(w678) -> ()
      n222 = Replace Substring(2:2 ("length (len. of substring)"), 3:w694, 5:w697) -> (1:w692:string)  [unwired: 1 in, 1 out]
      n223 = local read "Receive_Unpacked_Data"() -> (w690:T1)
      n224 = Bundle By Name(cluster=w690, "Decode_Data"=w692, "Time_To_Decode"=w678) -> (w691:T1)
    }
    frame "Battery Off" {
    }
    frame "Battery Charge Control" {
    }
    frame "Read Battery Voltage" {
      # "Voltage (MSB_LSB *.0006*2)"
      # "RESPONSE\nLength Byte:\t0x0D\nOpcode Byte:\t0x21\nSource Byte:\t0x00\nStatus Byte:\t0x80\nSub-opcode Byte:\t0x42\nData Byte 1:\t0x75: Attribute MSB\nData Byte 2:\t0x30: Attribute LSB\nData Byte 3:\t0x57: Attribute is Word ('W') value\nData Byte 4:\t0x01\nData Byte 5:\t0xXX: Battery Voltage MSB\nData Byte 6:\t0xXX: Battery Voltage LSB\nData Byte 7:\t0xFF: Packet Termination\nData Byte 8:\t0xFF: Packet Termination\nChecksum High Byte:\t0xXX\nChecksum Low Byte:\t0xXX"
      n225 = Array Subset(array=w716, index=0, length=15) -> (w715:u8[])
    }
    frame "RSM - SE4500 - GetPDM Calibration" {
      n226 = Index Array(array=w725, index=14) -> (element=w751:u8)
      n227 = Index Array(array=w725, index=16) -> (element=w744:u8)
      n228 = Index Array(array=w725, index=13) -> (element=w752:u8)
      n229 = Index Array(array=w725, index=15) -> (element=w745:u8)
      n230 = Index Array(array=w725, index=18) -> (element=w737:u8)
      n231 = Index Array(array=w725, index=20) -> (element=w731:u8)
      n232 = Index Array(array=w725, index=17) -> (element=w738:u8)
      n233 = Index Array(array=w725, index=19) -> (element=w732:u8)
      n234 = Join Numbers(hi=w751, lo=w752) -> ((hi.lo)=w724:u16)
      n235 = Join Numbers(hi=w744, lo=w745) -> ((hi.lo)=w721:u16)
      n236 = Join Numbers(hi=w737, lo=w738) -> ((hi.lo)=w722:u16)
      n237 = Join Numbers(hi=w731, lo=w732) -> ((hi.lo)=w723:u16)
      n238 = Number To Decimal String(number=w724, width (-)=i16 4) -> (decimal integer string=w750:string)
      n239 = Number To Decimal String(number=w721, width (-)=i16 4) -> (decimal integer string=w743:string)
      n240 = Number To Decimal String(number=w722, width (-)=i16 4) -> (decimal integer string=w736:string)
      n241 = Number To Decimal String(number=w723, width (-)=i16 4) -> (decimal integer string=w730:string)
      n242 = local read "Receive_Unpacked_Data"() -> (w748:T1)
      n243 = Bundle By Name(cluster=w748, "Response_String_1"=w750) -> (w741:T1)
      n244 = Bundle By Name(cluster=w741, "Response_String_2"=w743) -> (w728:T1)
      n245 = Bundle By Name(cluster=w728, "Response_String_3"=w736) -> (w727:T1)
      n246 = Bundle By Name(cluster=w727, "Response_String_4"=w730) -> (w726:T1)
    }
    frame "RSM - SE4500 - GetPDM-Z Calibration" {
      n247 = Index Array(array=w761, index=14) -> (element=w787:u8)
      n248 = Index Array(array=w761, index=16) -> (element=w780:u8)
      n249 = Index Array(array=w761, index=13) -> (element=w788:u8)
      n250 = Index Array(array=w761, index=15) -> (element=w781:u8)
      n251 = Index Array(array=w761, index=22) -> (element=w773:u8)
      n252 = Index Array(array=w761, index=24) -> (element=w767:u8)
      n253 = Index Array(array=w761, index=21) -> (element=w774:u8)
      n254 = Index Array(array=w761, index=23) -> (element=w768:u8)
      n255 = Join Numbers(hi=w787, lo=w788) -> ((hi.lo)=w760:u16)
      n256 = Join Numbers(hi=w780, lo=w781) -> ((hi.lo)=w757:u16)
      n257 = Join Numbers(hi=w773, lo=w774) -> ((hi.lo)=w758:u16)
      n258 = Join Numbers(hi=w767, lo=w768) -> ((hi.lo)=w759:u16)
      n259 = Number To Decimal String(number=w760, width (-)=i16 4) -> (decimal integer string=w786:string)
      n260 = Number To Decimal String(number=w757, width (-)=i16 4) -> (decimal integer string=w779:string)
      n261 = Number To Decimal String(number=w758, width (-)=i16 4) -> (decimal integer string=w772:string)
      n262 = Number To Decimal String(number=w759, width (-)=i16 4) -> (decimal integer string=w766:string)
      n263 = local read "Receive_Unpacked_Data"() -> (w784:T1)
      n264 = Bundle By Name(cluster=w784, "Response_String_1"=w786) -> (w777:T1)
      n265 = Bundle By Name(cluster=w777, "Response_String_2"=w779) -> (w764:T1)
      n266 = Bundle By Name(cluster=w764, "Response_String_3"=w772) -> (w763:T1)
      n267 = Bundle By Name(cluster=w763, "Response_String_4"=w766) -> (w762:T1)
    }
    frame "Get Object Sensor Value" {
      n268 = Index Array(array=w797, index=5) -> (element=w796:u8)
      n269 = Index Array(array=w797, index=6) -> (element=w795:u8)
      n270 = Number To Hexadecimal String(1:i16 2 ("width (-)"), 2:w796) -> (0:w804:string)
      n271 = Number To Hexadecimal String(1:i16 2 ("width (-)"), 2:w795) -> (0:w800:string)
      n272 = local read "Receive_Unpacked_Data"() -> (w802:T1)
      n273 = Bundle By Name(cluster=w802, "Response_String_1"=w804) -> (w798:T1)
      n274 = Bundle By Name(cluster=w798, "Response_String_2"=w800) -> (w793:T1)
    }
    frame "Read Object Sensor Calibration Value" {
      n275 = Index Array(array=w811, index=9) -> (element=w810:u8)
      n276 = Index Array(array=w811, index=10) -> (element=w809:u8)
      n277 = Number To Hexadecimal String(1:i16 2 ("width (-)"), 2:w810) -> (0:w818:string)
      n278 = Number To Hexadecimal String(1:i16 2 ("width (-)"), 2:w809) -> (0:w814:string)
      n279 = local read "Receive_Unpacked_Data"() -> (w816:T1)
      n280 = Bundle By Name(cluster=w816, "Response_String_1"=w818) -> (w812:T1)
      n281 = Bundle By Name(cluster=w812, "Response_String_2"=w814) -> (w807:T1)
    }
    frame "Store Object Sensor Calibration Value" {
    }
    frame "Read Battery Temperature" {
      # "RESPONSE\nLength Byte:\t0x0D\nOpcode Byte:\t0x21\nSource Byte:\t0x00\nStatus Byte:\t0x80\nSub-opcode Byte:\t0x42\nData Byte 1:\t0x75: Attribute MSB\nData Byte 2:\t0x31: Attribute LSB\nData Byte 3:\t0x57: Attribute is Word ('W') value\nData Byte 4:\t0x01\nData Byte 5:\t0xXX: Battery Temperature MSB\nData Byte 6:\t0xXX: Battery Temperature LSB\nData Byte 7:\t0xFF: Packet Termination\nData Byte 8:\t0xFF: Packet Termination\nChecksum High Byte:\t0xXX\nChecksum Low Byte:\t0xXX"
      n282 = Array Subset(array=w827, index=0, length=15) -> (w826:u8[])
    }
    frame "Software Version" {
      n283 = Array Subset(array=w837, index=32, length=16) -> (w834:u8[])
      n284 = Array Subset(array=w837, index=13, length=16) -> (w840:u8[])
      n285 = Byte Array To String(unsigned byte array=w840) -> (string=w833:string)
      n286 = Byte Array To String(unsigned byte array=w834) -> (string=w832:string)
      n287 = Concatenate Strings(w833, "  " ("string"), w832) -> (w830:string)
      n288 = local read "Receive_Unpacked_Data"() -> (w839:T1)
      n289 = Bundle By Name(cluster=w839, "Code_Revision"=w830) -> (w838:T1)
    }
    frame "StoreFeatureSet" {
    }
    frame "ReadFeatureSet" {
      # "Feature Set Responce:\n0x0C, 0x21, 0x00, 0x00, 0x42, 0x02, 0xC2,0x42,0x01,\n\t\t\t\t\t\t\t\t\t\t\t  \t\t\t  0xff, //FEATURE-SET\n\t\t\t\t\t\t\t\t\t\t\t\t\t\t  0xff,0xff, // packet termination\n\t\t\t\t\t\t\t\t\t\t\t\t\t\t  0x00, 0x00}; //checksum"
      n290 = Array Subset(array=w851, index=9, length=1) -> (w848:u8[])
    }
    frame "Store Model Number" {
    }
    frame "Read Model Number" {
      n291 = Array Subset(array=w861, index=13, length=18) -> (w859:u8[])
      n292 = Byte Array To String(unsigned byte array=w859) -> (string=w860:string)
      n293 = local read "Receive_Unpacked_Data"() -> (w858:T1)
      n294 = Bundle By Name(cluster=w858, "Response_String_1"=w860) -> (w857:T1)
    }
    frame "Store Manufacturing Date" {
      n295 = Get Date/Time In Seconds() -> (seconds since 1Jan1904=w872:timestamp)
      n296 = Format Date/Time String(time format string (%c)="%d%b%y", seconds (now)=w872, UTC format=FALSE) -> (date/time string=w869:string)
      n297 = To Upper Case(1:w869) -> (0:w866:string)
      n298 = local read "Receive_Unpacked_Data"() -> (w868:T1)
      n299 = Bundle By Name(cluster=w868, "Response_String_1"=w866) -> (w867:T1)
    }
    frame "Read Manufacturing Date" {
      n300 = Array Subset(array=w880, index=13, length=7) -> (w877:u8[])
      n301 = Byte Array To String(unsigned byte array=w877) -> (string=w879:string)
      n302 = local read "Receive_Unpacked_Data"() -> (w876:T1)
      n303 = Bundle By Name(cluster=w876, "Response_String_1"=w879) -> (w878:T1)
    }
    frame "Store Service Date" {
    }
    frame "Read Service Date" {
      n304 = Array Subset(array=w892, index=13, length=7) -> (w890:u8[])
      n305 = Byte Array To String(unsigned byte array=w890) -> (string=w891:string)
      n306 = local read "Receive_Unpacked_Data"() -> (w889:T1)
      n307 = Bundle By Name(cluster=w889, "Response_String_1"=w891) -> (w888:T1)
    }
    frame "Store Serial Number" {
    }
    frame "Read Serial Number" {
      n308 = Array Subset(array=w904, index=13, length=16) -> (w900:u8[])
      n309 = Byte Array To String(unsigned byte array=w900) -> (string=w903:string)
      n310 = local read "Receive_Unpacked_Data"() -> (w901:T1)
      n311 = Bundle By Name(cluster=w901, "Response_String_1"=w903) -> (w902:T1)
    }
    frame "Query Paired Address" {
      # "Cradle BT Address"
      # "Pair Status\n0x00: Unpaired \n0x01: Paired"
      n312 = Array Subset(array=w912, index=6, length=6) -> (w915:u8[])
      n313 = Array Subset(array=w912, index=5, length=1) -> (w910:u8[])
      n314 = local read "Receive_Unpacked_Data"() -> (w909:T1)
      n315 = Byte Array To String(unsigned byte array=w915) -> (string=w916:string)
      n316 = Bundle By Name(cluster=w909, "Response_String_1"=w916) -> (w911:T1)
    }
    frame "Pairing Status" {
      # "Pairing Status\n0x00: Cradle is not paired\n0x01: Cradle is paired"
      n317 = Empty Array?(array=w921) -> (empty?=w922:bool)
      n318 = case shown="False" w922 {
        tunnel: w921 -> [w927 _]
        tunnel: [w926 w933] -> w923
        frame False {
          n319 = Array Subset(array=w927, index=5, length=1) -> (w926:u8[])
        }
        frame True {
          # "If empty, init array and set its values to zero."
          n320 = To Unsigned Byte Integer(number=u8 0) -> (unsigned 8bit integer=w931:u8)
          n321 = Initialize Array(w931, 1 ("dimension size")) -> (w933:u8[])
        }
      }
    }
    frame "Read GUID" {
      n322 = Array Subset(array=w937, index=5, length=32) -> (w936:u8[])
      n323 = Byte Array To String(unsigned byte array=w936) -> (string=w940:string)
      n324 = local read "Receive_Unpacked_Data"() -> (w935:T1)
      n325 = Bundle By Name(cluster=w935, "Response_String_1"=w940) -> (w934:T1)
    }
    frame "Cable Auto ID" {
    }
    frame "Store RSM 627" {
    }
    frame "Store GUID " {
    }
    frame "Hall Effect switch" {
      n326 = Empty Array?(array=w953) -> (empty?=w954:bool)
      n327 = case shown="True" w954 {
        tunnel: w953 -> [w960 _]
        tunnel: [w959 w966] -> w952
        frame False {
          n328 = Array Subset(array=w960, index=5, length=1) -> (w959:u8[])
        }
        frame True {
          # "If empty, init array and set its values to zero."
          n329 = To Unsigned Byte Integer(number=u8 0) -> (unsigned 8bit integer=w964:u8)
          n330 = Initialize Array(w964, 1 ("dimension size")) -> (w966:u8[])
        }
      }
      n331 = Array Subset(array=w953, index=5, length=1) -> ()  [unwired: 1 out]
    }
    frame "Read RSM 627" {
    }
  }
  "error out" <- w11
  "Receive_buffer" <- w12
  "VISA resource name OUT" <- w13
  "Receive_Unpacked_Data" <- w9
  "TimeToDecode" <- u16 0 ("TimeToDecode")
